vi "变量读取.vi"() -> (0 "错误输出":errorcluster)   [LabVIEW 2016, in "中水三立SQL数据传输.lvlib"]
uses:
  <vilib>/Utility/config.llb/NI_LVConfig.lvlib
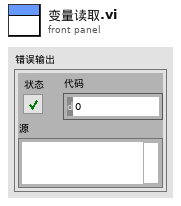
[diagram p1: front panel]
types:
  T1 = typedef "NI_LVConfig.lvlib/Config Data RefNum.ctl" = refnum<k1>
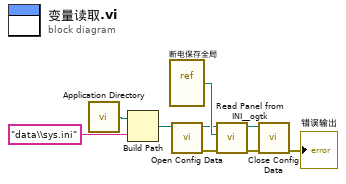
[diagram p0: block diagram]
diagram:
  n1 = call <vilib>:"Application Directory.vi"() -> ("Application Directory"=w5:path)
  n2 = Build Path(base path=w5, name or relative path="data\\sys.ini" ("名称或相对路径")) -> (appended path=w6:path)
  n3 = vi-ref "断电保存全局.vi"() -> (w8:refnum<vi>)
  n4 = call <vilib>:"Open Config Data.vi"("configuration file path"=w6) -> ("error out"=w2:errorcluster, "refnum"=w3:T1)  [unwired: 8 in, 1 out]
  n5 = call <userlib>:"Read Panel from INI__ogtk.vi"("error in (no error)"=w2, "VI ref"=w8, "refnum"=w3) -> ("error out"=w1:errorcluster, "refnum out"=w4:T1)  [unwired: 7 in]
  n6 = call <vilib>:"Close Config Data.vi"("error in (no error)"=w1, "refnum"=w4) -> ("error out"=→"错误输出":errorcluster)  [unwired: 8 in, 1 out]
